vi "泵温度校准配置.vi"() -> ()   [LabVIEW 2016]
uses:
  <vilib>/Utility/miscctls.llb/LVPointTypeDef.ctl
panel:
  in  "关闭":bool
  in  "偏心轮校准簇":T1={"复位"=FALSE, "进纯水"=FALSE, "停止"=FALSE, "液体重量"=60, "偏心轮校准"=FALSE}
  in  "温度校准簇":T2={"进纯水"=FALSE, "排液"=FALSE, "停止 2"=FALSE, "开始加热"=FALSE, "温度值"=115.0, "温度校准"=FALSE}
  # "偏心轮、温度校准"
  # "输入实际液体重量:"
  # "g"
  # "温度:"
  # "℃"
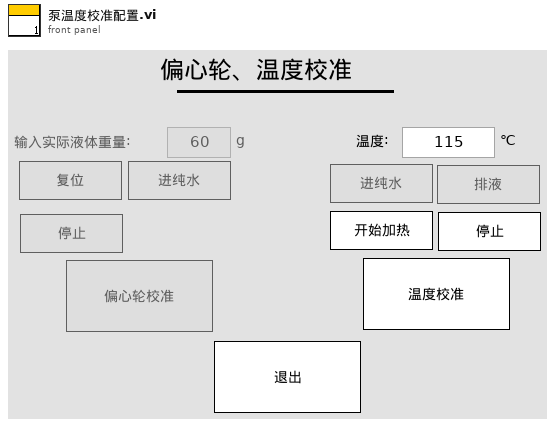
[diagram p1: front panel]
types:
  T1 = cluster{"复位":bool, "进纯水":bool, "停止":bool, "液体重量":u16, "偏心轮校准":bool}
  T2 = cluster{"进纯水":bool, "排液":bool, "停止 2":bool, "开始加热":bool, "温度值":dbl, "温度校准":bool}
  T3 = enum8{"Enabled", "Disabled", "Disabled and Grayed Out"}
  T4 = typedef "LVPointTypeDef.ctl" = cluster{"Horizontal":i16, "Vertical":i16}
  T5 = cluster{"泵类型":u8, "阀数量":u8, "纯水通道":u8, "废液通道":u8, "进样速度":u16, "出样速度":u16, "滴定速度":u16, "注射泵保温温度L":u8, "注射泵保温温度H":u8, "注射泵加热超时时间":u16, "是否存在液位检测板":u16, "A值告警下限值":u16, "A值告警上限值":u16, "B值告警下限值":u16, "B值告警上限值":u16, "AB跨度告警值":u16, "阀配置:":u8, "滴定等待时间":u16, "滴定吸光度斜率":dbl}
  T6 = cluster{"系统时间":timestamp, "工作状态":u16, "测量模式":enum16{"待机", "连续模式", "周期模式", "定点模式", "受控模式", "手动模式"}, "告警代码":u16, "故障代码":u16, "日志代码":u16, "软件版本":u16, "测量间隔":u16, "消解实时温度":dbl, "校准间隔（天）":u16, "校准间隔（时）":u16, "周期测量时间（23_16）":u16, "周期测量时间（15_0）":u16, "清洗周期（次数）":u16, "运行模式":u16, "自动校准状态":u16, "自动清洗状态":u16}
  T7 = cluster{"偏心轮校准参数":dbl, "运行速度(修改需要重启)":u16, "加热温度(校准参数) ":dbl, "告警温度":dbl, "加热超时时间:(单位/秒)":dbl, "K p":dbl, "K i":dbl, "K d":dbl, "ILimitUp":dbl, "ILimitDown":dbl}
  T8 = cluster{"检出限":dbl, "测量精度":dbl, "上限":dbl, "下限":dbl, "阈值（低->高）":dbl, "阈值（高->低）":dbl}
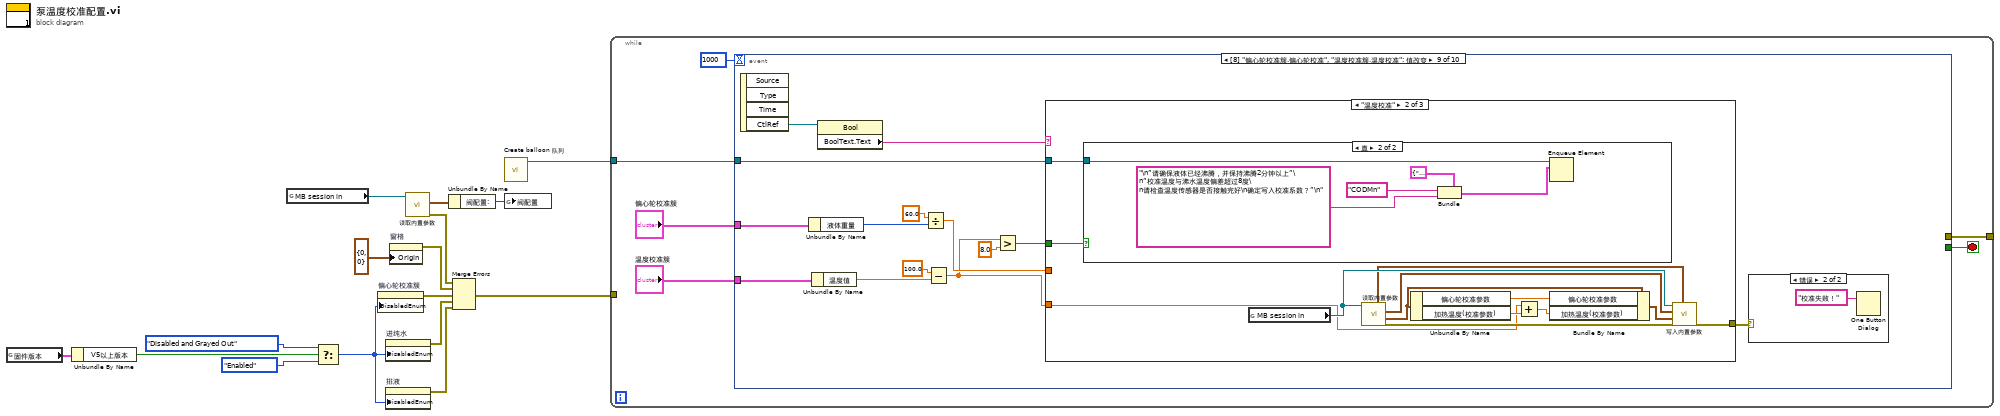
[diagram p0: block diagram]
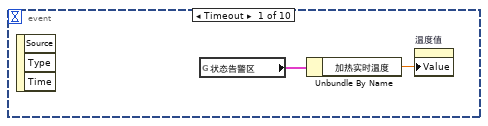
[diagram p2: hidden frame]
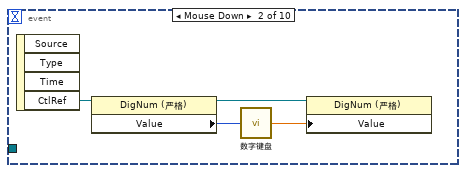
[diagram p3: hidden frame]
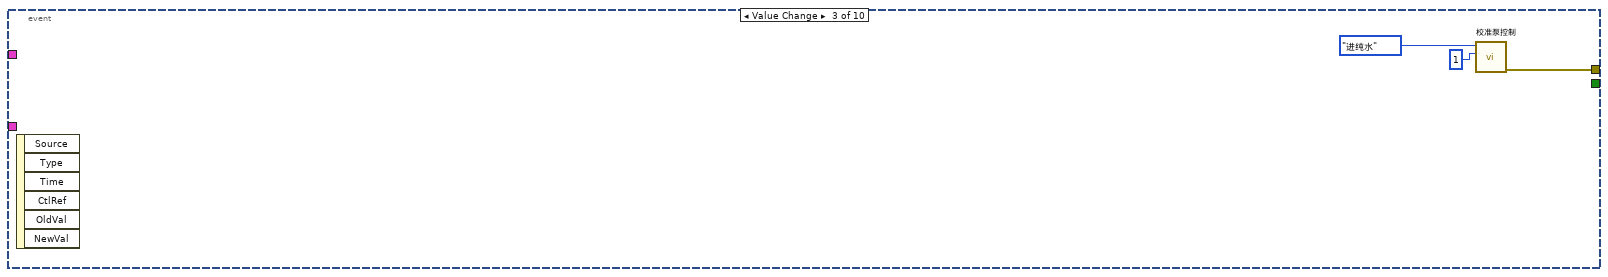
[diagram p4: hidden frame]
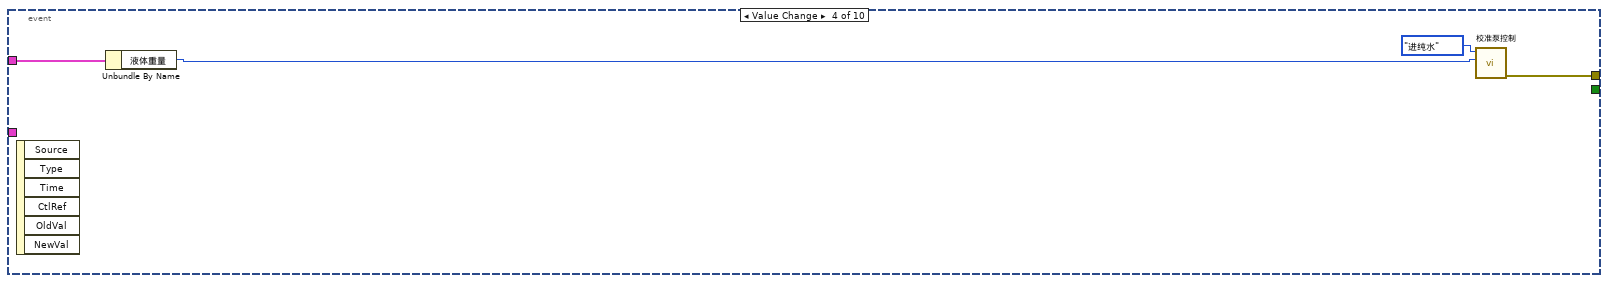
[diagram p5: hidden frame]
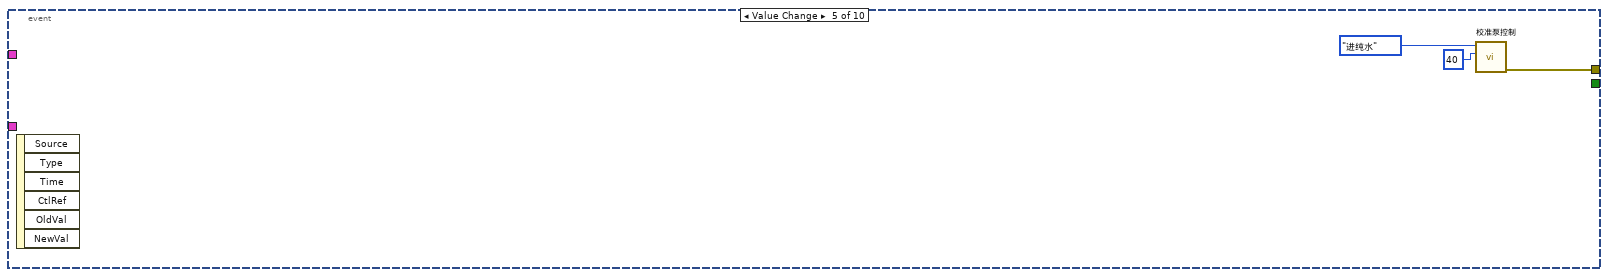
[diagram p6: hidden frame]
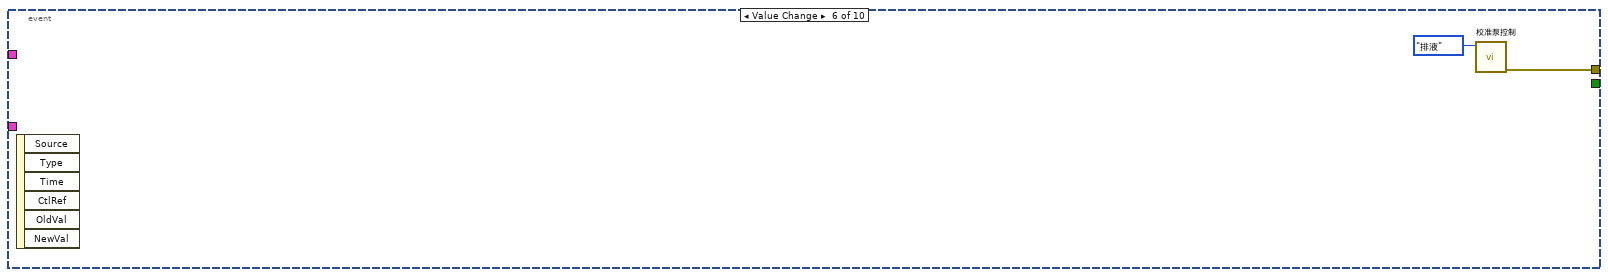
[diagram p7: hidden frame]
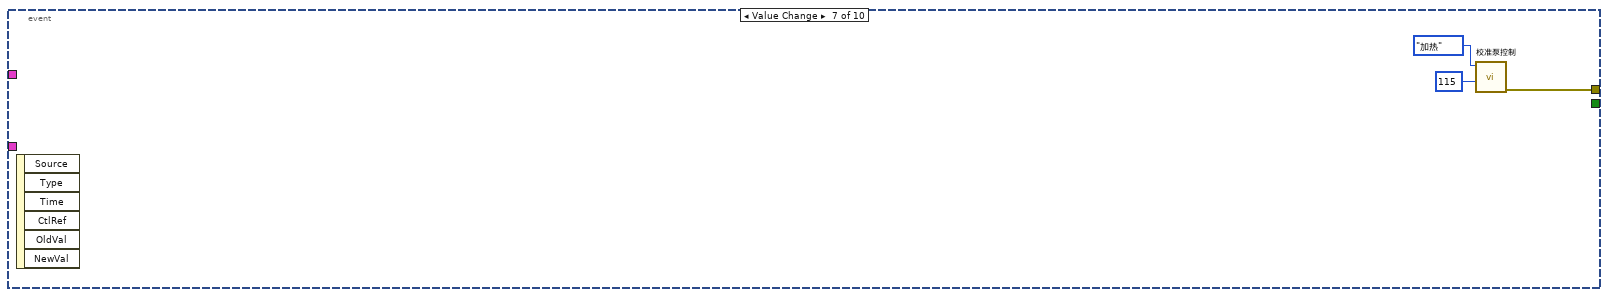
[diagram p8: hidden frame]
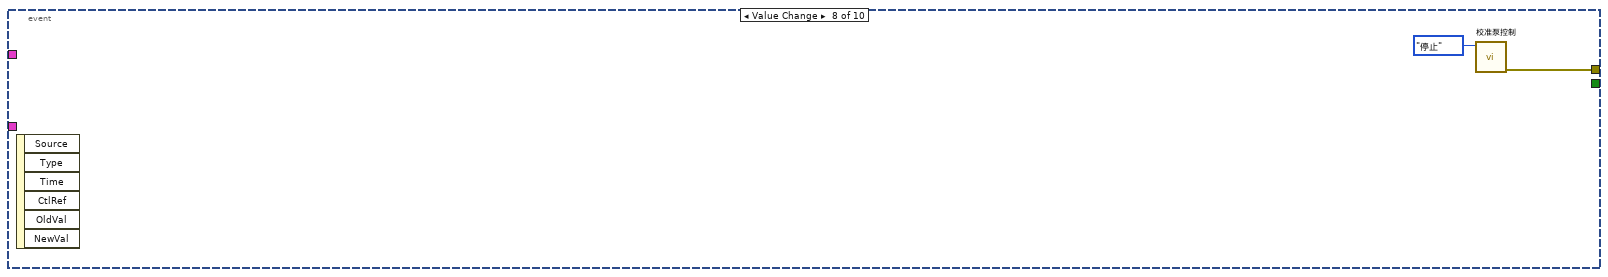
[diagram p9: hidden frame]
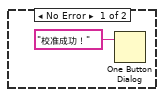
[diagram p10: hidden frame]
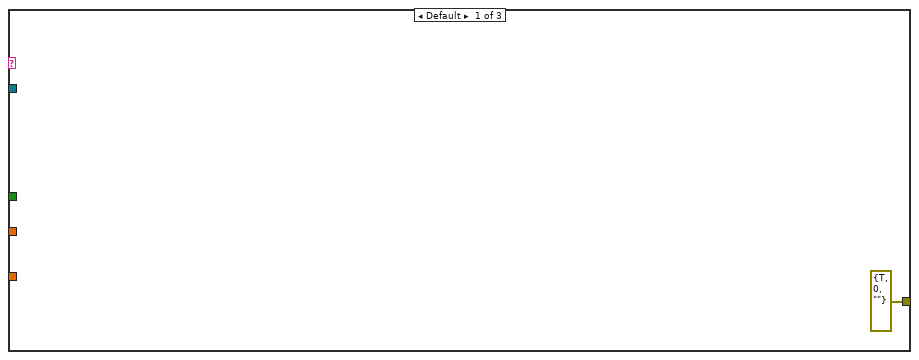
[diagram p11: hidden frame]
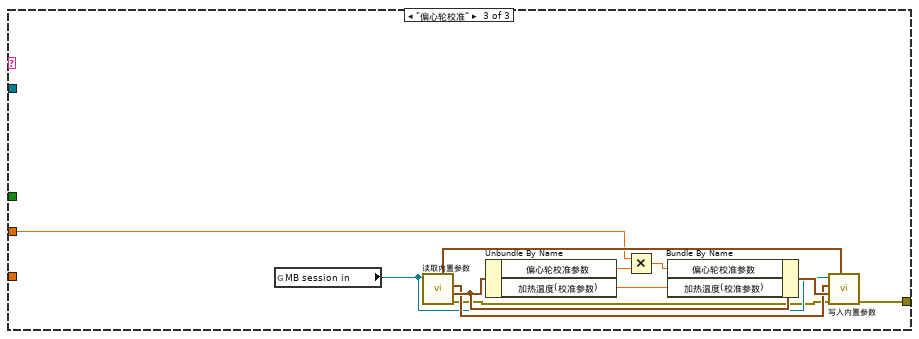
[diagram p13: hidden frame]
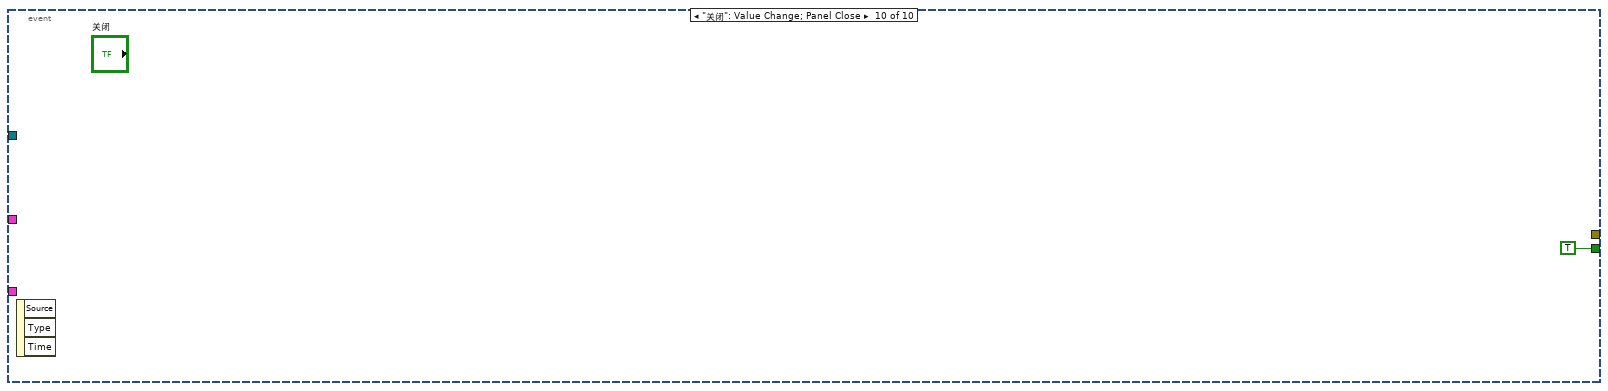
[diagram p14: hidden frame]
diagram:
  n1 = global read "VAR挥发酚全局变量.vi" "固件版本"() -> (w2:cluster{"V5以上版本":bool, "版本号":dbl})
  n2 = Unbundle By Name(w2) -> ("V5以上版本"=w1:bool)
  n3 = global read "VAR挥发酚全局变量.vi" "MB session in"() -> (w14:refnum<class "MB_Master.lvclass">)
  n4 = Select(t=T3."Disabled and Grayed Out" ("禁用"), s=w1, f=T3."Enabled" ("禁用")) -> (s? t:f=w9:T3)
  n5 = property on="偏心轮校准簇" class="Clust"("DisabledEnum"=w9) -> (error out=w6:errorcluster)  [unwired: 2 in, 1 out]
  n6 = property on="进纯水" class="Bool"("DisabledEnum"=w9) -> (error out=w5:errorcluster)  [unwired: 2 in, 1 out]
  n7 = property on="排液" class="Bool"("DisabledEnum"=w9) -> (error out=w4:errorcluster)  [unwired: 2 in, 1 out]
  n8 = property on="窗格" class="Pane"("Origin"=T4 {"Horizontal"=0, "Vertical"=0} ("原点")) -> (error out=w7:errorcluster)  [unwired: 2 in, 1 out]
  n9 = call "读取内置参数.vi"("MB session in"=w14) -> ("error out"=w8:errorcluster, "外设配置"=w13:T5)  [unwired: 6 in, 3 out]
  n10 = Unbundle By Name(w13) -> ("阀配置:"=w12:u8)
  n11 = Merge Errors(w8, w7, w6, w5, w4) -> (w3:errorcluster)
  n12 = call "Create balloon 队列.vi"() -> ("队列输出"=w15:refnum<queue>)  [unwired: 11 in]
  n13 = global write "挥发酚断电保存全局变量.vi" "阀配置"(w12) -> ()
  n14 = while {
    tunnel: [w21] -> _
    tunnel: w15 -> [w19]
    tunnel: w3 -> [_]
    stop <- w22 stop-if-true
    n15 = event shown="[8] \"偏心轮校准簇.偏心轮校准\", \"温度校准簇.温度校准\": 值改变" {
      selector: _ -> [_ _ _ _ _ _ _ _ _ _]
      dyn-events: _ -> [_ _ _ _ _ _ _ _ _ _]
      timeout: 1000 -> [_ _ _ _ _ _ _ _ _ _]
      tunnel: [_ _ _ _ _ _ _ _ _ TRUE] -> w22
      tunnel: "偏心轮校准簇" -> [_ _ _ w34 _ _ _ _ w59 _]
      tunnel: [_ _ w30 w35 w38 w40 w43 w45 _ _] -> w21
      tunnel: "温度校准簇" -> [_ _ _ _ _ _ _ _ w46 _]
      tunnel: w19 -> [_ _ _ _ _ _ _ _ w48 _]
      event Timeout {
        n16 = event-data() -> ()  [unwired: 1 in, 3 out]
        n17 = global read "VAR挥发酚全局变量.vi" "状态告警区"() -> (w24:T6)
        n18 = Unbundle By Name(w24) -> ("加热实时温度"=w23:sgl)
        n19 = property on="温度值" class="DigNum (严格)"("Value"=w23) -> ()  [unwired: 2 in, 2 out]
      }
      event "偏心轮校准簇.液体重量": Mouse Down {
        n20 = event-data() -> ("CtlRef"=w25:refnum<vi>)  [unwired: 1 in, 3 out]
        n21 = property class="DigNum (严格)"(reference=w25) -> (reference out=w27:refnum<vi>, "Value"=w28:u16)  [unwired: 1 in, 1 out]
        n22 = call "数字键盘.vi"("OldNumber"=w28) -> ("NewNumber"=w26:dbl)
        n23 = property class="DigNum (严格)"(reference=w27, "Value"=w26) -> ()  [unwired: 1 in, 2 out]
      }
      event "偏心轮校准簇.复位": Value Change {
        n24 = event-data() -> ()  [unwired: 1 in, 6 out]
        n25 = call "校准泵控制.vi"("偏心轮"=u16 1, "枚举"=enum16{"进水样", "进纯水", "排液", "加热", "停止"}."进纯水") -> ("错误输出"=w30:errorcluster)  [unwired: 9 in]
      }
      event "偏心轮校准簇.进纯水": Value Change {
        n26 = event-data() -> ()  [unwired: 1 in, 6 out]
        n27 = Unbundle By Name(w34) -> ("液体重量"=w33:u16)
        n28 = call "校准泵控制.vi"("偏心轮"=w33, "枚举"=enum16{"进水样", "进纯水", "排液", "加热", "停止"}."进纯水") -> ("错误输出"=w35:errorcluster)  [unwired: 9 in]
      }
      event "温度校准簇.进纯水": Value Change {
        n29 = event-data() -> ()  [unwired: 1 in, 6 out]
        n30 = call "校准泵控制.vi"("偏心轮"=u16 40, "枚举"=enum16{"进水样", "进纯水", "排液", "加热", "停止"}."进纯水") -> ("错误输出"=w38:errorcluster)  [unwired: 9 in]
      }
      event "温度校准簇.排液": Value Change {
        n31 = event-data() -> ()  [unwired: 1 in, 6 out]
        n32 = call "校准泵控制.vi"("枚举"=enum16{"进水样", "进纯水", "排液", "加热", "停止"}."排液") -> ("错误输出"=w40:errorcluster)  [unwired: 10 in]
      }
      event "温度校准簇.开始加热": Value Change {
        n33 = event-data() -> ()  [unwired: 1 in, 6 out]
        n34 = call "校准泵控制.vi"("摄氏度"=u16 115, "枚举"=enum16{"进水样", "进纯水", "排液", "加热", "停止"}."加热") -> ("错误输出"=w43:errorcluster)  [unwired: 9 in]
      }
      event "温度校准簇.停止 2", "偏心轮校准簇.停止": Value Change {
        n35 = event-data() -> ()  [unwired: 1 in, 6 out]
        n36 = call "校准泵控制.vi"("枚举"=enum16{"进水样", "进纯水", "排液", "加热", "停止"}."停止") -> ("错误输出"=w45:errorcluster)  [unwired: 10 in]
      }
      event "偏心轮校准簇.偏心轮校准", "温度校准簇.温度校准": Value Change {
        n37 = event-data() -> ("CtlRef"=w53:refnum<vi>)  [unwired: 1 in, 3 out]
        n38 = Unbundle By Name(w59) -> ("液体重量"=w57:u16)
        n39 = Unbundle By Name(w46) -> ("温度值"=w55:dbl)
        n40 = property class="Bool"(reference=w53) -> ("BoolText.Text"=w50:string)  [unwired: 1 in, 2 out]
        n41 = Divide(x=60.0, y=w57) -> (x/y=w52:dbl)
        n42 = Subtract(x=100.0, y=w55) -> (x-y=w51:dbl)
        n43 = Greater?(x=w51, y=8.0) -> (0:w49:bool)
        n44 = case shown="\"温度校准\"" w50 {
          tunnel: w52 -> [_ _ w83]
          tunnel: w51 -> [_ w65 _]
          tunnel: w49 -> [_ w67 _]
          tunnel: w48 -> [_ w66 _]
          tunnel: [errorcluster {"status"=TRUE, "code"=0, "source"=""} ("error out") w63 w81] -> w47
          frame Default {
          }
          frame "温度校准" {
            n45 = case shown="真" w67 {
              tunnel: w66 -> [_ w80]
              frame False {
              }
              frame True {
                n46 = Bundle(cluster=cluster{"Title":string, "Body":string} {"Title"="", "Body"=""} ("元素"), "Title"="CODMn", "Body"="\n”请确保液体已经沸腾，并保持沸腾2分钟以上”\n”校准温度与沸水温度偏差超过8度\n请检查温度传感器是否接触完好\n确定写入校准系数？”\n") -> (w76:cluster{"Title":string, "Body":string})
                n47 = Enqueue Element(queue=w80, element=w76) -> ()  [unwired: 2 in, 3 out]
              }
            }
            n48 = global read "VAR挥发酚全局变量.vi" "MB session in"() -> (w70:refnum<class "MB_Master.lvclass">)
            n49 = call "读取内置参数.vi"("MB session in"=w70) -> ("error out"=w68:errorcluster, "float"=w72:T7, "外设配置"=w71:T5, "量程参数读取"=w69:T8)  [unwired: 6 in, 1 out]
            n50 = Unbundle By Name(w72) -> ("偏心轮校准参数"=w64:dbl, "加热温度(校准参数)"=w74:dbl)
            n51 = Add(x=w65, y=w74) -> (x+y=w75:dbl)
            n52 = Bundle By Name(cluster=w72, "偏心轮校准参数"=w64, "加热温度(校准参数)"=w75) -> (w73:T7)
            n53 = call "写入内置参数.vi"("量程参数读取"=w69, "error in (no error)"=w68, "float"=w73, "外设配置"=w71, "MB session in"=w70) -> ("error out"=w63:errorcluster)  [unwired: 5 in, 1 out]
          }
          frame "偏心轮校准" {
            n54 = global read "VAR挥发酚全局变量.vi" "MB session in"() -> (w86:refnum<class "MB_Master.lvclass">)
            n55 = call "读取内置参数.vi"("MB session in"=w86) -> ("error out"=w84:errorcluster, "float"=w88:T7, "外设配置"=w87:T5, "量程参数读取"=w85:T8)  [unwired: 6 in, 1 out]
            n56 = Unbundle By Name(w88) -> ("偏心轮校准参数"=w90:dbl, "加热温度(校准参数)"=w82:dbl)
            n57 = Multiply(x=w83, y=w90) -> (x*y=w91:dbl)
            n58 = Bundle By Name(cluster=w88, "偏心轮校准参数"=w91, "加热温度(校准参数)"=w82) -> (w89:T7)
            n59 = call "写入内置参数.vi"("量程参数读取"=w85, "error in (no error)"=w84, "float"=w89, "外设配置"=w87, "MB session in"=w86) -> ("error out"=w81:errorcluster)  [unwired: 5 in, 1 out]
          }
        }
        n60 = case shown="错误" w47 {
          frame No Error {
            n61 = One Button Dialog(message="校准成功！" ("消息")) -> ()  [unwired: 1 in, 1 out]
          }
          frame Error {
            n62 = One Button Dialog(message="校准失败！" ("消息")) -> ()  [unwired: 1 in, 1 out]
          }
        }
      }
      event "关闭": Value Change; Panel Close {
        n63 = event-data() -> ()  [unwired: 1 in, 3 out]
      }
    }
  }
